vi "number_ROIs.vi"(8 "error in":errorcluster, 11 "Display State In":T2={"current frame index"=0, "number of images"=0, "ROI (frames)"={"ROI"=[]}, "control refs"={"frame"=refnum, "image"=refnum, "saveROIsButton"=refnum, "loadImageSwitch"=refnum, "loadROIsSwitch"=refnum, "saveROIsSwitch"=refnum, "loadImagePath"=refnum, "loadROIPath"=refnum, "redraw"=refnum}, "calibration"={"x"=0.0, "y"=0.0, "x unit"=enum."um", "y unit"=enum."um"}, "xpaths"={"x offset"="", "y offset"="", "z offset"=""}, "offset"=refnum, "XML description"="", "number of ROIs"=0.0, "ROI Tool Buttons Visible"={"Zoom Tool"=FALSE, "Selection Tool"=FALSE, "Pan Tool"=FALSE, "Point Tool"=FALSE, "Line Tool"=FALSE, "Rectangle Tool"=FALSE, "Rotated Rectangle Tool"=FALSE, "Polyline Tool"=FALSE, "Polygon Tool"=FALSE, "Freehand Tool"=FALSE, "Closed Freehand Tool"=FALSE, "Ellipse Tool"=FALSE, "Annulus Tool"=FALSE}, "ROI color"=0, "enable ROI numbering?"=FALSE, "selected path to save ROIs"=path "", "starting path"=path "", "array of overlays"=[], "pointCollection"=refnum, "ROImode"=enum."none", "selected point ID"=1.0, "point radius"=0, "point colours"=[], "PlotAreaSize"={"Width"=0, "Height"=0}, "last action"=enum."not specified"} {"array of overlays"."overlay size" min=1}) -> (0 "error out":errorcluster, 3 "Display State Out":T2={"current frame index"=0, "number of images"=0, "ROI (frames)"={"ROI"=[]}, "control refs"={"frame"=refnum, "image"=refnum, "saveROIsButton"=refnum, "loadImageSwitch"=refnum, "loadROIsSwitch"=refnum, "saveROIsSwitch"=refnum, "loadImagePath"=refnum, "loadROIPath"=refnum, "redraw"=refnum}, "calibration"={"x"=0.0, "y"=0.0, "x unit"=enum."um", "y unit"=enum."um"}, "xpaths"={"x offset"="", "y offset"="", "z offset"=""}, "offset"=refnum, "XML description"="", "number of ROIs"=0.0, "ROI Tool Buttons Visible"={"Zoom Tool"=FALSE, "Selection Tool"=FALSE, "Pan Tool"=FALSE, "Point Tool"=FALSE, "Line Tool"=FALSE, "Rectangle Tool"=FALSE, "Rotated Rectangle Tool"=FALSE, "Polyline Tool"=FALSE, "Polygon Tool"=FALSE, "Freehand Tool"=FALSE, "Closed Freehand Tool"=FALSE, "Ellipse Tool"=FALSE, "Annulus Tool"=FALSE}, "ROI color"=0, "enable ROI numbering?"=FALSE, "selected path to save ROIs"=path "", "starting path"=path "", "array of overlays"=[], "pointCollection"=refnum, "ROImode"=enum."none", "selected point ID"=1.0, "point radius"=0, "point colours"=[], "PlotAreaSize"={"Width"=0, "Height"=0}, "last action"=enum."not specified"} {"array of overlays"."overlay size" min=1})   [LabVIEW 2010, in "XImage.xctl"]
uses:
  XImage.xctl
  state.ctl
  classes/SpaceVector/SpaceVector/SpaceVector.lvclass
  classes/PointCollection/PointCollection/PointCollection.lvclass
  ROI_frames_cluster.ctl
  control_refs_cluster.ctl
  calibration_cluster.ctl
  enumerations/unit.ctl
  xpath_cluster.ctl
  overlays_cluster.ctl
  ROI_mode_enum.ctl
  last_action_enum.ctl
  <vilib>/vision/Image Controls.llb/IMAQ Image.ctl
  classes/Image/Image/Image.lvclass
panel:
  in  "Font, Size & Style":T1={"Desired Font (Application)"=enum."Application Font", "[User-specified Font]"={"Font Name"="", "Size"=12, "Strikeout?"=FALSE, "Italic?"=FALSE, "Underline?"=FALSE, "Outline?"=FALSE, "Shadow?"=FALSE, "Bold?"=FALSE, "Rotation Angle"=0.0}, "Horizontal Alignment"=0, "Vertical Alignment"=0} {"Horizontal Alignment" items=["Left", "Center", "Right"]; "Vertical Alignment" items=["Bottom", "Top", "Baseline"]}
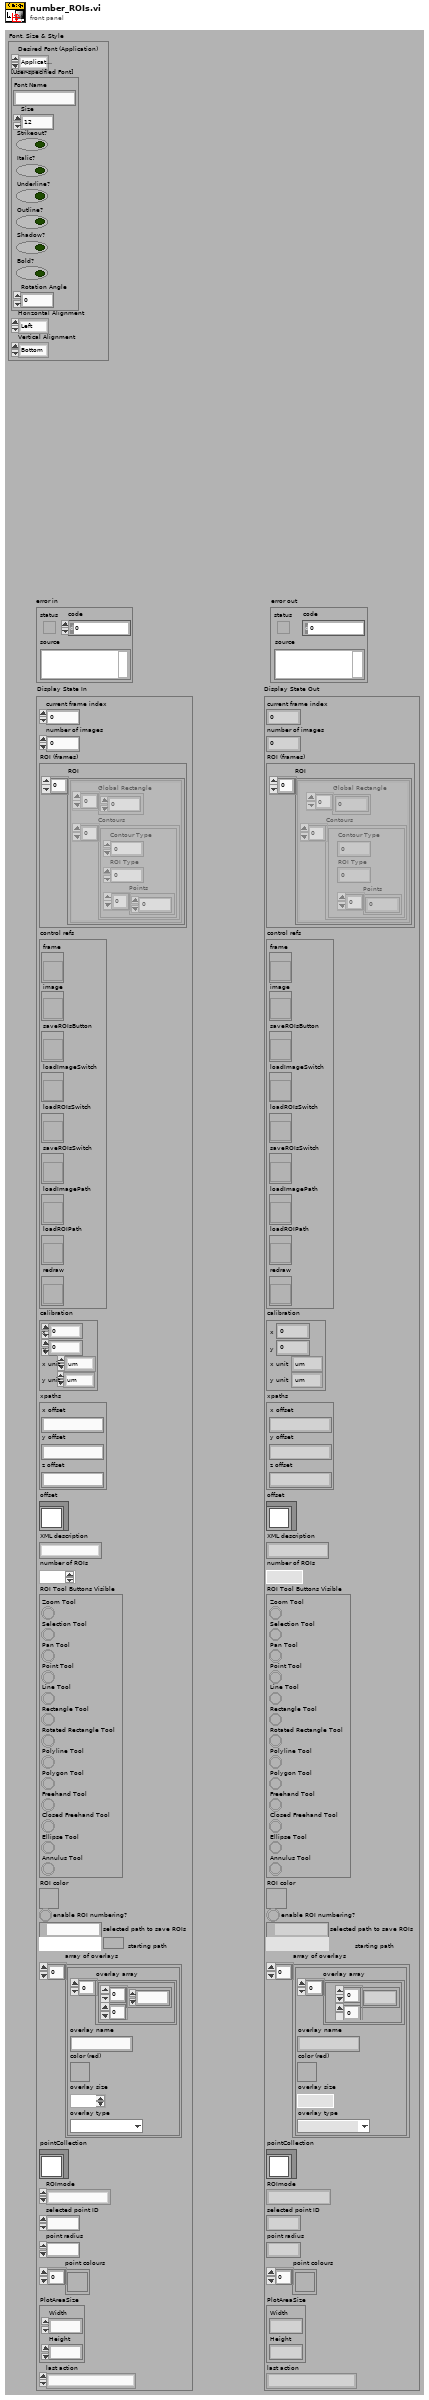
[diagram p1: front panel]
types:
  T1 = cluster{"Desired Font (Application)":enum16{"User-specified Font", "Application Font", "System Font", "Dialog Font"}, "[User-specified Font]":cluster{"Font Name":string, "Size":i16, "Strikeout?":bool, "Italic?":bool, "Underline?":bool, "Outline?":bool, "Shadow?":bool, "Bold?":bool, "Rotation Angle":dbl}, "Horizontal Alignment":i16, "Vertical Alignment":i16}
  T2 = typedef "XImage.xctl/state.ctl" = cluster{"current frame index":i32, "number of images":i32, "ROI (frames)":T3, "control refs":T4, "calibration":T5, "xpaths":T7, "offset":refnum<class "SpaceVector.lvclass">, "XML description":string, "number of ROIs":dbl, "ROI Tool Buttons Visible":cluster{"Zoom Tool":bool, "Selection Tool":bool, "Pan Tool":bool, "Point Tool":bool, "Line Tool":bool, "Rectangle Tool":bool, "Rotated Rectangle Tool":bool, "Polyline Tool":bool, "Polygon Tool":bool, "Freehand Tool":bool, "Closed Freehand Tool":bool, "Ellipse Tool":bool, "Annulus Tool":bool}, "ROI color":u32, "enable ROI numbering?":bool, "selected path to save ROIs":path, "starting path":path, "array of overlays":T8[], "pointCollection":refnum<class "PointCollection.lvclass">, "ROImode":T9, "selected point ID":dbl, "point radius":i32, "point colours":u32[], "PlotAreaSize":cluster{"Width":u32, "Height":u32}, "last action":T10}
  T3 = typedef "XImage.xctl/ROI_frames_cluster.ctl" = cluster{"ROI":cluster{"Global Rectangle":i32[], "Contours":cluster{"Contour Type":u32, "ROI Type":u32, "Points":i32[]}[]}[]}
  T4 = typedef "XImage.xctl/control_refs_cluster.ctl" = cluster{"frame":refnum<vi>, "image":refnum<vi>, "saveROIsButton":refnum<vi>, "loadImageSwitch":refnum<vi>, "loadROIsSwitch":refnum<vi>, "saveROIsSwitch":refnum<vi>, "loadImagePath":refnum<vi>, "loadROIPath":refnum<vi>, "redraw":refnum<vi>}
  T5 = typedef "XImage.xctl/calibration_cluster.ctl" = cluster{"x":dbl, "y":dbl, "x unit":T6, "y unit":T6}
  T6 = typedef "Image.lvclass/unit.ctl" = enum16{"um", "s"}
  T7 = typedef "XImage.xctl/xpath_cluster.ctl" = cluster{"x offset":string, "y offset":string, "z offset":string}
  T8 = typedef "XImage.xctl/overlays_cluster.ctl" = cluster{"overlay array":cluster{i32[][]}[], "overlay name":string, "color (red)":u32, "overlay size":i32, "overlay type":enum16{"crosshair", "circle"}}
  T9 = typedef "XImage.xctl/ROI_mode_enum.ctl" = enum16{"none", "IMAQROIs", "PointCollection"}
  T10 = typedef "XImage.xctl/last_action_enum.ctl" = enum16{"not specified", "image loaded", "frame changed", "ROIs changed"}
  T11 = typedef "IMAQ Image.ctl" = refnum<image>
  T12 = cluster{"Global Rectangle":i32[], "Contours":cluster{"Contour Type":u32, "ROI Type":u32, "Points":i32[]}[]}[]
  T13 = cluster{"Contour Type":u32, "ROI Type":u32, "Points":i32[]}[]
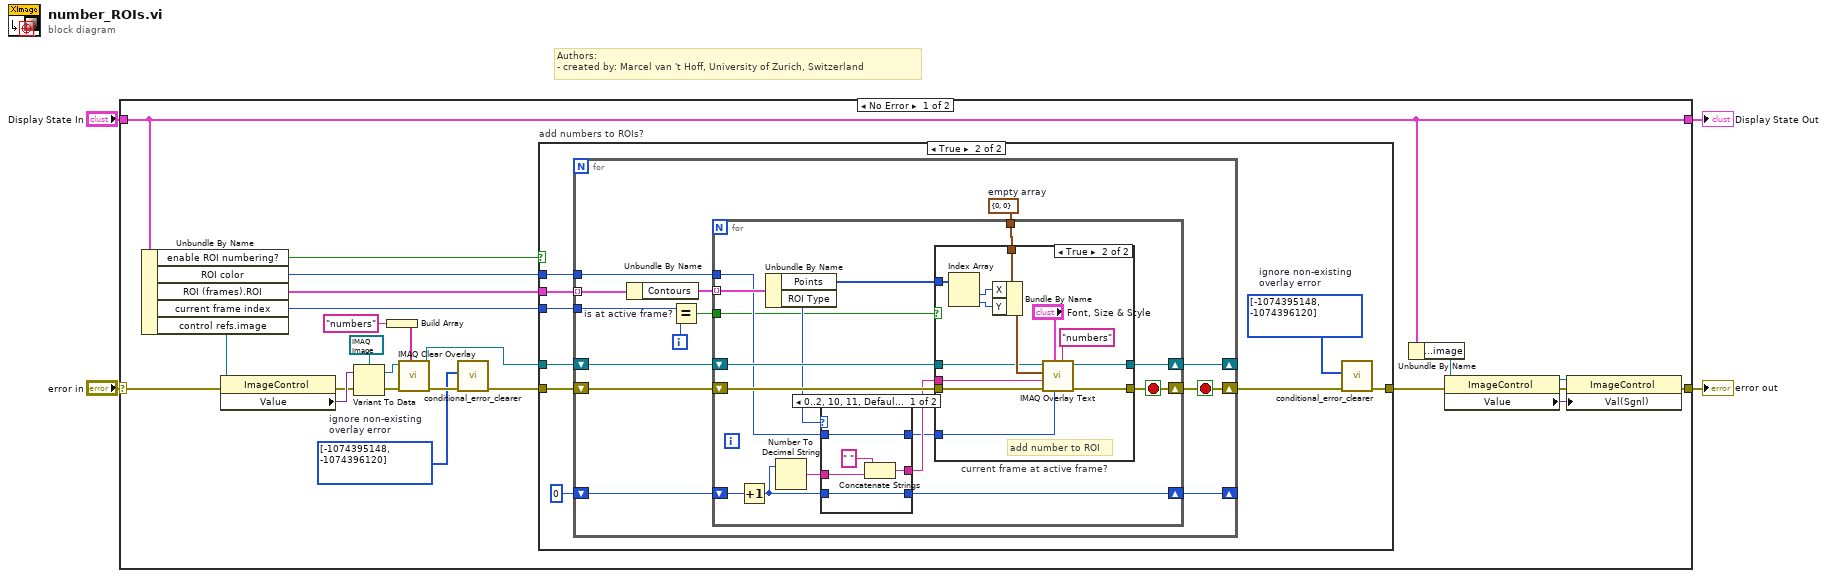
[diagram p0: block diagram]
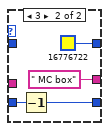
[diagram p4: hidden frame]
diagram:
  # "Authors: \n- created by: Marcel van 't Hoff, University of Zurich, Switzerland"
  n1 = case shown="No Error" "error in" {
    selector: "error in" -> [w27 w93]
    tunnel: [w7 w93] -> w3
    tunnel: "Display State In" -> [w11 w92]
    tunnel: [w11 w92] -> w1
    frame No Error {
      w12 = i32[] [-1074395148, -1074396120]  # ignore non-existing overlay error
      n2 = Unbundle By Name(w11) -> ("enable ROI numbering?"=w18:bool, "ROI color"=w17:u32, "ROI (frames).ROI"=w16:T12, "current frame index"=w15:i32, "control refs.image"=w28:refnum<vi>)
      n3 = property class="ImageControl"(reference=w28, error in=w27) -> (error out=w24:errorcluster, "Value"=w26:variant)  [unwired: 1 out]
      n4 = Variant To Data(error in=w24, Variant=w26, type=T11 refnum ("New Image")) -> (error out=w20:errorcluster, data=w21:T11)
      n5 = Build Array("numbers" ("String")) -> (w22:string[])
      n6 = call "IMAQ Clear Overlay"("Groups"=w22, "error in (no error)"=w20, "Image"=w21) -> ("error out"=w14:errorcluster, "Image Out"=w19:T11)  [unwired: 7 in]
      n7 = call "conditional_error_clearer.vi"("error in (no error)"=w14, "array of clearable error codes"=w12) -> ("error out"=w13:errorcluster)  [unwired: 9 in]
      n8 = case "add numbers to ROIs?" shown="True" w18 {
        tunnel: w13 -> [w29 w38]
        tunnel: w19 -> [_ w37]
        tunnel: w16 -> [_ w36]
        tunnel: [w29 w31] -> w6
        tunnel: w17 -> [_ w35]
        tunnel: w15 -> [_ w33]
        frame False {
        }
        frame True {
          w30 = i32[] [-1074395148, -1074396120]  # ignore non-existing overlay error
          n9 = for {
            tunnel: w36 -> [w47] mode=indexing
            tunnel: w35 -> [w48]
            shift-right: [w40] -> w32
            shift-left: w38 -> [w51]
            shift-right: [w44] -> _
            shift-left: 0 ("x+1") -> [w45]
            tunnel: w33 -> [w43]
            shift-right: [w39] -> _
            shift-left: w37 -> [w50]
            i -> [w42]
            stop <- w40 stop-if-true
            w49 = cluster{"X":i32, "Y":i32} {"X"=0, "Y"=0}  # empty array
            n10 = Unbundle By Name(w47) -> ("Contours"=w46:T13)
            n11 = Equal? "is at active frame?"(x=w43, y=w42) -> (x = y?=w41:bool)
            n12 = for {
              tunnel: w46 -> [w67] mode=indexing
              tunnel: w49 -> [w65]
              shift-right: [w61] -> w40
              shift-left: w51 -> [w62]
              shift-right: [w63] -> w39
              shift-left: w50 -> [w64]
              shift-right: [w56] -> w44
              shift-left: w45 -> [w55]
              tunnel: w48 -> [w53]
              tunnel: w41 -> [w52]
              stop <- w61 stop-if-true
              n13 = Increment(x=w55) -> (x+1=w54:i32)
              n14 = Unbundle By Name(w67) -> ("Points"=w66:i32[], "ROI Type"=w60:u32)
              n15 = Number To Decimal String(number=w54) -> (decimal integer string=w59:string)  [unwired: 1 in]
              n16 = case shown="0..2, 10, 11, Default" w60 {
                tunnel: w59 -> [w87 _]
                tunnel: [w85 " MC box" ("string")] -> w58
                tunnel: [w83 u32 16776722 ("Text Color (black)")] -> w57
                tunnel: [w84 w88] -> w56
                tunnel: w54 -> [w84 w89]
                tunnel: w53 -> [w83 _]
                frame 0..2, 10, 11, Default {
                  n17 = Concatenate Strings(" " ("string"), w87) -> (w85:string)
                }
                frame 3 {
                  n18 = Decrement(x=w89) -> (x-1=w88:i32)
                }
              }
              n19 = case "current frame at active frame?" shown="True" w52 {
                tunnel: w66 -> [_ w82]
                tunnel: w65 -> [_ w79]
                tunnel: w64 -> [w68 w77]
                tunnel: [w68 w76] -> w63
                tunnel: w62 -> [w69 w75]
                tunnel: [w69 w74] -> w61
                tunnel: w58 -> [_ w72]
                tunnel: w57 -> [_ w71]
                frame False {
                }
                frame True {
                  # "add number to ROI"
                  n20 = Index Array(array=w82) -> (element #1=w81:i32, element #2=w80:i32)  [unwired: 2 in]
                  n21 = Bundle By Name(cluster=w79, "X"=w81, "Y"=w80) -> (w78:cluster{"X":i32, "Y":i32})
                  n22 = call "IMAQ Overlay Text"("Group"="numbers", "Text Color (black)"=w71, "Font, Size & Style"="Font, Size & Style", "error in (no error)"=w75, "String"=w72, "Origin"=w78, "Image"=w77) -> ("error out"=w74:errorcluster, "Image Out"=w76:T11)  [unwired: 3 in]
                }
              }
            }
          }
          n23 = call "conditional_error_clearer.vi"("error in (no error)"=w32, "array of clearable error codes"=w30) -> ("error out"=w31:errorcluster)  [unwired: 9 in]
        }
      }
      n24 = Unbundle By Name(w11) -> ("control refs.image"=w10:refnum<vi>)
      n25 = property class="ImageControl"(reference=w10, error in=w6) -> (reference out=w9:refnum<vi>, error out=w8:errorcluster, "Value"=w5:variant)
      n26 = property class="ImageControl"(reference=w9, error in=w8, "Val(Sgnl)"=w5) -> (error out=w7:errorcluster)  [unwired: 1 out]
    }
    frame Error {
    }
  }
  "error out" <- w3
  "Display State Out" <- w1
